vi "GExplorer_Queue_GEA2.vi"(0 "Output String":string, 11 "error in (no error)":errorcluster) -> (15 "error out":errorcluster)   [LabVIEW 2014]
uses:
  typedefs/GExplorer_Data_Cluster.ctl
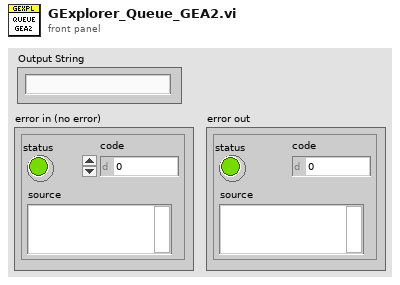
[diagram p1: front panel]
types:
  T1 = typedef "GExplorer_Data_Cluster.ctl" = cluster{"Data":variant, "State":enum16{"Add to Log", "Clear", "Shutdown"}}
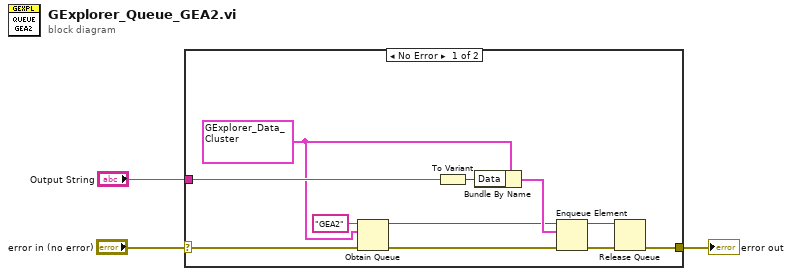
[diagram p0: block diagram]
diagram:
  n1 = case shown="No Error" "error in (no error)" {
    selector: "error in (no error)" -> [w11 w15]
    tunnel: [w5 w15] -> w3
    tunnel: "Output String" -> [w12 _]
    frame No Error {
      w4 = T1 {"Data"=variant, "State"=enum."Add to Log"} ("Data")
      n2 = Obtain Queue(name (unnamed)="GEA2", element data type=w4, error in (no error)=w11) -> (queue out=w9:refnum<queue>, error out=w10:errorcluster)  [unwired: 2 in, 1 out]
      n3 = To Variant(anything=w12) -> (Variant=w13:variant)
      n4 = Bundle By Name(cluster=w4, "Data"=w13) -> (w14:T1)
      n5 = Enqueue Element(queue=w9, element=w14, error in (no error)=w10) -> (queue out=w6:refnum<queue>, error out=w7:errorcluster)  [unwired: 1 in, 1 out]
      n6 = Release Queue(queue=w6, error in (no error)=w7) -> (error out=w5:errorcluster)  [unwired: 1 in, 2 out]
    }
    frame Error {
    }
  }
  "error out" <- w3
